vi "SetBitfiledValue(Bool).vi"(8 "error in (no error)":errorcluster, 9 "bitfield value":bool, 10 "bitfield caps":T1={"offset"=0, "size"=0, "signed?"=TRUE}, 11 "original value":u64 format="%.0x") -> (0 "error out":errorcluster, 3 "update value":u64 format="%.0x")   [LabVIEW 2018, in "Bitfield.lvlib"]
uses:
  Bitfield.lvlib
  BitfieldCaps.ctl
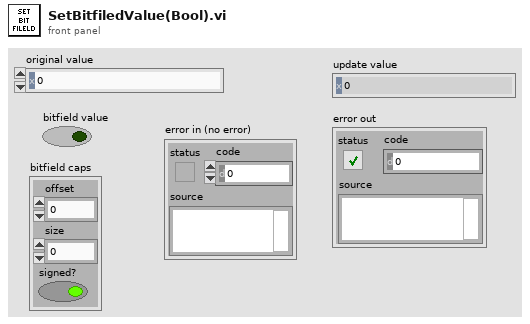
[diagram p1: front panel]
types:
  T1 = typedef "Bitfield.lvlib/BitfieldCaps.ctl" = cluster{"offset":i32, "size":i32, "signed?":bool}
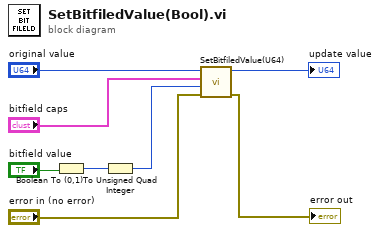
[diagram p0: block diagram]
diagram:
  n1 = Boolean To (0,1)(Boolean="bitfield value") -> (0, 1=w2:i16)
  n2 = To Unsigned Quad Integer(1:w2) -> (0:w1:u64)
  n3 = call "SetBitfiledValue(U64).vi"("error in (no error)"="error in (no error)", "bitfield value"=w1, "bitfield caps"="bitfield caps", "original value"="original value") -> ("error out"=→"error out":errorcluster, "update value"=→"update value":u64)  [unwired: 6 in]
